vi "Inst.KH7008.getShuntResistor.vi"(8 "error in (no error)":errorcluster, 11 "Inst.Krohn-Hite-7008 in":refnum<class "Inst.Krohn-Hite-7008.lvclass">) -> (0 "error out":errorcluster, 2 "ShuntResistor":string, 3 "Inst.Krohn-Hite-7008 out":refnum<class "Inst.Krohn-Hite-7008.lvclass">)   [LabVIEW 2019, in "Inst.KH7008.lvlib" / "Inst.Krohn-Hite-7008.lvclass"]
doc: "Returns the installed shunt resistor set"
uses:
  Inst.Krohn-Hite-7008.lvclass
  Typedefs/Inst.KH7008.Commands--Enum.ctl
  Typedefs/getShuntResistorResponse--Cluster.ctl
  1fdc1f3d-332e-4594-8a59-3c61ed5849a6.vi
  1fdc1f3d-332e-4594-8a59-3c61ed5849a6.vi/6461b58b-b02c-486d-a597-2279dba98f21.vi
  1fdc1f3d-332e-4594-8a59-3c61ed5849a6.vi/deb96b58-bc0e-4b79-bcdf-b1bc8e4b7beb.vi
  <vilib>/Utility/Data Type/Get Type Information.vi
  <vilib>/JDP Science/JSONtext/JSON text to Variant.vi
  <vilib>/JDP Science/JSONtext/LVClass Serializer/JSONtext LVClass Serializer.lvclass
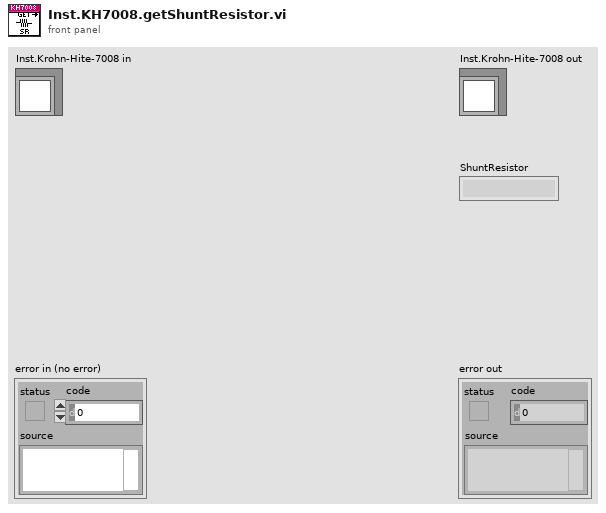
[diagram p1: front panel]
types:
  T1 = typedef "Inst.KH7008.lvlib/Inst.Krohn-Hite-7008.lvclass/getShuntResistorResponse--Cluster.ctl" = cluster{"ShuntResistor":string}
  T2 = typedef "Inst.KH7008.lvlib/Inst.Krohn-Hite-7008.lvclass/Inst.KH7008.Commands--Enum.ctl" = enum16{"getChannel", "getAllChannels", "setChannel", "setAllChannels", "getShuntResistor"}
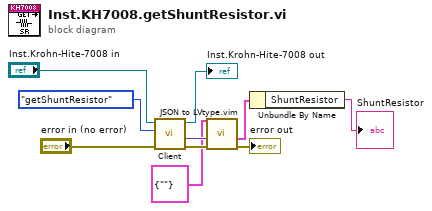
[diagram p0: block diagram]
diagram:
  n1 = call-dynamic "Client.vi"("error in (no error)"="error in (no error)", "Command in"=Inst.KH7008.Commands--Enum."getShuntResistor" ("publicCommands"), "Instrument in"="Inst.Krohn-Hite-7008 in") -> ("error out"=w5:errorcluster, "Data out"=w6:variant, "Instrument out"=→"Inst.Krohn-Hite-7008 out":refnum<class "Inst.Krohn-Hite-7008.lvclass">)  [unwired: 5 in, 1 out]
  n2 = call "JSON to LVtype.vim"("type"=T1 {"ShuntResistor"=""} ("getShuntResistor"), "error in (no error)"=w5, "JSON Data in"=w6) -> ("error out"=→"error out":errorcluster, "Data out"=w2:T1)  [unwired: 7 in]
  n3 = Unbundle By Name(w2) -> ("ShuntResistor"=→"ShuntResistor":string)
